vi "LJLogUD process data.vi"(6 "Disable Scaling":bool, 9 "Channel Config":T1={"# Channels"=4, "+Ch"=["0", "1", "2", "3", "4", "5", "6", "7"], "-Ch (U3)"=["31", "31", "31", "31", "31", "31", "31", "31"], "Ranges (UE9)"=[0, 0, 0, 0, 0, 0, 0, 0], "Scaling Equation"=["y=v0", "y=v1", "y=v2", "y=v3", "y=v4", "y=v5", "y=v6", "y=v7"]} {"Ranges (UE9)" items=["LJ_rgBIP5V", "LJ_rgUNI5V", "LJ_rgUNI2P5V", "LJ_rgUNI1P25V", "LJ_rgUNIP625V"]}, 11 "Voltages":dbl[][](array[numeric]) format="%.3f") -> (2 "Volts,Scaled Averages":dbl[][](array[numeric]) format="%.3f", 3 "Scaled Data":dbl[][](array[numeric]) format="%.3f")   [LabVIEW 2020]
uses:
  <vilib>/Analysis/NI_AALBase.lvlib
  <vilib>/Analysis/baseanly.llb/Mean (DBL).vi
panel:
  out "ms":u32
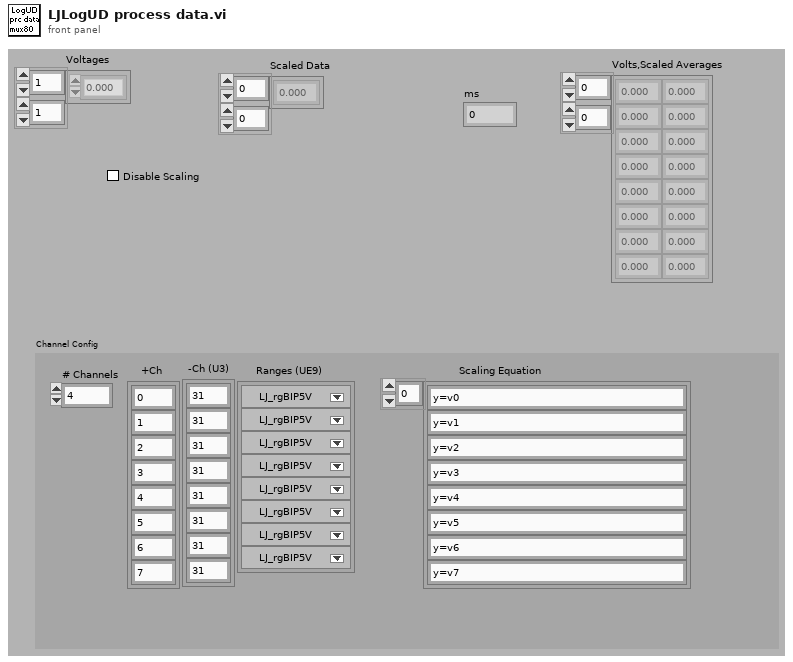
[diagram p1: front panel]
types:
  T1 = cluster{"# Channels":i32, "+Ch":string[], "-Ch (U3)":string[], "Ranges (UE9)":u16[], "Scaling Equation":string[]}
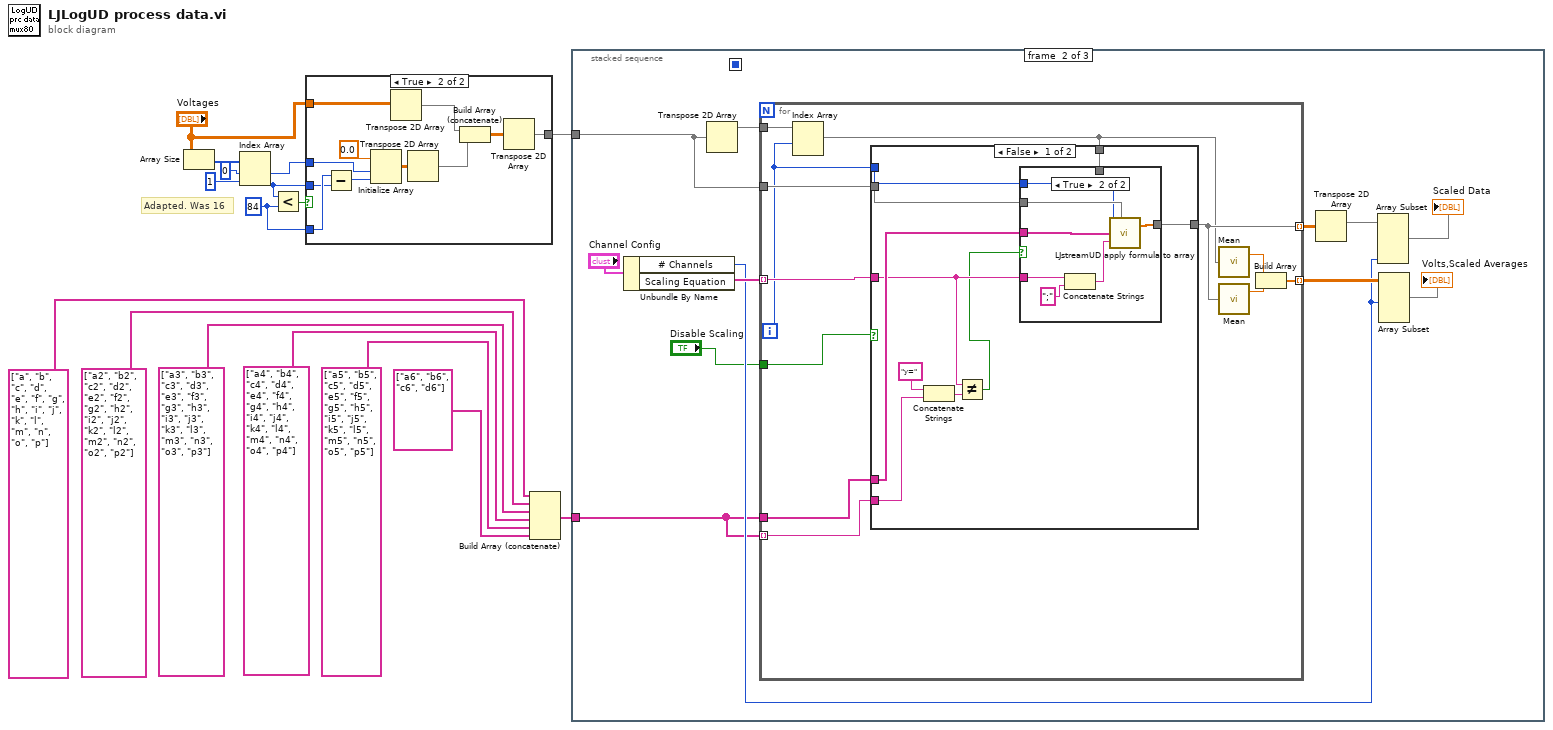
[diagram p0: block diagram]
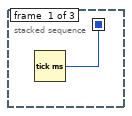
[diagram p3: hidden frame]
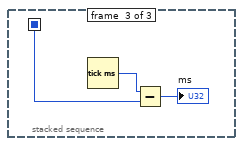
[diagram p6: hidden frame]
diagram:
  w12 = 84 ("y")
  # "Adapted. Was 16"
  n1 = Array Size(array="Voltages") -> (size(s)=w14:i32[])
  n2 = Index Array(array=w14, index #1=0 ("Index"), index #2=1 ("Index")) -> (element #1=w10:i32, element #2=w11:i32)
  n3 = Less?(x=w11, y=w12) -> (x < y?=w13:bool)
  n4 = case shown="True" w13 {
    tunnel: w12 -> [_ w28]
    tunnel: w11 -> [_ w27]
    tunnel: w10 -> [_ w26]
    tunnel: "Voltages" -> [w17 w23]
    tunnel: [w17 w20] -> w8
    frame False {
    }
    frame True {
      n5 = Subtract(x=w28, y=w27) -> (x-y=w25:i32)
      n6 = Initialize Array(0.0, w26, w25) -> (w19:dbl[][])
      n7 = Transpose 2D Array(2D array=w23) -> (transposed array=w22:dbl[][])
      n8 = Transpose 2D Array(2D array=w19) -> (transposed array=w18:dbl[][])
      n9 = Build Array (concatenate)(w22, w18) -> (w21:dbl[][])
      n10 = Transpose 2D Array(2D array=w21) -> (transposed array=w20:dbl[][])
    }
  }
  n11 = Build Array (concatenate)(string[] ["a", "b", "c", "d", "e", "f", "g", "h", "i", "j", "k", "l", "m", "n", "o", "p"], string[] ["a2", "b2", "c2", "d2", "e2", "f2", "g2", "h2", "i2", "j2", "k2", "l2", "m2", "n2", "o2", "p2"], string[] ["a3", "b3", "c3", "d3", "e3", "f3", "g3", "h3", "i3", "j3", "k3", "l3", "m3", "n3", "o3", "p3"], string[] ["a4", "b4", "c4", "d4", "e4", "f4", "g4", "h4", "i4", "j4", "k4", "l4", "m4", "n4", "o4", "p4"], string[] ["a5", "b5", "c5", "d5", "e5", "f5", "g5", "h5", "i5", "j5", "k5", "l5", "m5", "n5", "o5", "p5"], string[] ["a6", "b6", "c6", "d6"]) -> (w7:string[])
  n12 = stacked-sequence {
    seq-local: [w29 _ _] -> [_ _ w74]
    tunnel: w8 -> [_ w37 _]
    tunnel: w7 -> [_ w31 _]
    frame #0 {
      n13 = Tick Count (ms)() -> (millisecond timer value=w29:u32)
    }
    frame #1 {
      n14 = Unbundle By Name("Channel Config") -> ("# Channels"=w32:i32, "Scaling Equation"=w38:string[])
      n15 = Transpose 2D Array(2D array=w37) -> (transposed array=w40:dbl[][])
      n16 = for {
        tunnel: w37 -> [w49]
        tunnel: w38 -> [w48] mode=indexing
        tunnel: [w50] -> w41 mode=indexing
        tunnel: [w51] -> w36 mode=indexing
        tunnel: w40 -> [w47]
        tunnel: w31 -> [w44]
        tunnel: w31 -> [w43] mode=indexing
        tunnel: "Disable Scaling" -> [w42]
        i -> [w45]
        n17 = Index Array(array=w47, index (row)=w45) -> (element=w46:dbl[])  [unwired: 1 in]
        n18 = case shown="False" w42 {
          tunnel: [w63 w72] -> w50
          tunnel: w49 -> [w62 _]
          tunnel: w48 -> [w57 _]
          tunnel: w46 -> [w54 w72]
          tunnel: w45 -> [w61 _]
          tunnel: w44 -> [w60 _]
          tunnel: w43 -> [w56 _]
          frame False {
            n19 = Concatenate Strings("y=", w56) -> (w58:string)
            n20 = Not Equal?(x=w57, y=w58) -> (x != y?=w55:bool)
            n21 = case shown="True" w55 {
              tunnel: [w64 w71] -> w63
              tunnel: w62 -> [_ w70]
              tunnel: w61 -> [_ w67]
              tunnel: w60 -> [_ w66]
              tunnel: w57 -> [_ w65]
              tunnel: w54 -> [w64 _]
              frame False {
              }
              frame True {
                n22 = Concatenate Strings(w65, ";" ("Substring")) -> (w69:string)
                n23 = call "LJstreamUD apply formula to array.vi"("Index"=w67, "Input Values"=w70, "Variables Input"=w66, "formula"=w69) -> ("Output Values"=w71:dbl[])  [unwired: 1 in, 1 out]
              }
            }
          }
          frame True {
          }
        }
        n24 = call-poly <vilib>:"Mean.vi"("X"=w46) -> ("mean"=w53:dbl)  [unwired: 1 out]
        n25 = call-poly <vilib>:"Mean.vi"("X"=w50) -> ("mean"=w52:dbl)  [unwired: 1 out]
        n26 = Build Array(w53, w52) -> (w51:dbl[])
      }
      n27 = Transpose 2D Array(2D array=w41) -> (transposed array=w34:dbl[][])
      n28 = Array Subset(array=w34, length (col)=w32) -> (→"Scaled Data":dbl[][])  [unwired: 3 in]
      n29 = Array Subset(array=w36, length (row)=w32) -> (→"Volts,Scaled Averages":dbl[][])  [unwired: 3 in]
    }
    frame #2 {
      n30 = Tick Count (ms)() -> (millisecond timer value=w75:u32)
      n31 = Subtract(x=w75, y=w74) -> (x-y=→"ms":u32)
    }
  }
